vi "file operation select.vi"(1 "File in":refnum<class "File.lvclass">) -> (0 "Operation":T1=enum."Moving")   [LabVIEW 2023, in "File Classes.lvlib" / "File.lvclass"]
uses:
  File.lvclass
  Controls/file operation enum.ctl
  File.lvclass/File.ctl
  File Classes.lvlib
panel:
  # "Called in multiple places"
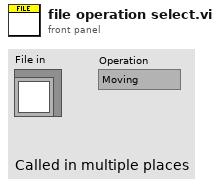
[diagram p1: front panel]
types:
  T1 = typedef "File Classes.lvlib/file operation enum.ctl" = enum16{"Copying", "Moving", "Deleting", "Skipped", "Renaming"}
  T2 = typedef "File Classes.lvlib/file operation settings mode.ctl" = enum16{"Copy Files", "Move Files", "Rename Files"}
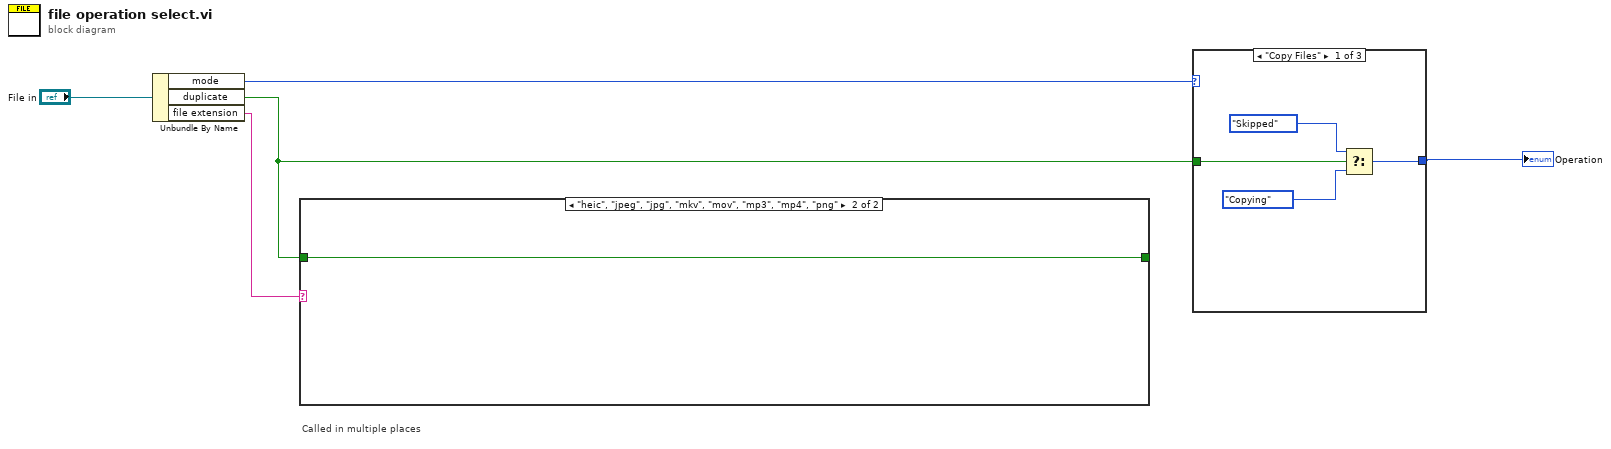
[diagram p0: block diagram]
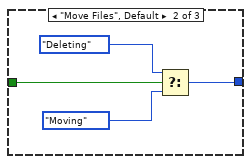
[diagram p2: hidden frame]
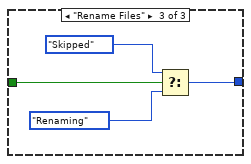
[diagram p3: hidden frame]
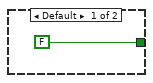
[diagram p4: hidden frame]
diagram:
  # "Called in multiple places"
  n1 = Unbundle By Name("File in") -> ("mode"=w3:T2, "duplicate"=w1:bool, "file extension"=w4:string)
  n2 = case shown="\"heic\", \"jpeg\", \"jpg\", \"mkv\", \"mov\", \"mp3\", \"mp4\", \"png\"" w4 {
    tunnel: [FALSE ("duplicate") w7] -> _
    tunnel: w1 -> [_ w7]
    frame Default {
    }
    frame "heic", "jpeg", "jpg", "mkv", "mov", "mp3", "mp4", "png" {
    }
  }
  n3 = case shown="\"Copy Files\"" w3 {
    tunnel: w1 -> [w11 w15 w19]
    tunnel: [w10 w14 w18] -> w2
    frame "Copy Files" {
      n4 = Select(t=file_operation_enum."Skipped" ("Operation"), s=w11, f=file_operation_enum."Copying" ("Operation")) -> (s? t:f=w10:T1)
    }
    frame "Move Files", Default {
      n5 = Select(t=file_operation_enum."Deleting" ("Operation"), s=w15, f=file_operation_enum."Moving" ("Operation")) -> (s? t:f=w14:T1)
    }
    frame "Rename Files" {
      n6 = Select(t=file_operation_enum."Skipped" ("Operation"), s=w19, f=file_operation_enum."Renaming" ("Operation")) -> (s? t:f=w18:T1)
    }
  }
  "Operation" <- w2
